vi "Configure Trigger.vi"(0 "VISA resource name":refnum<visa-resource-name>, 5 "Trigger Sequence (1: Output 1)":i32(ring)=1 items=["Output"=1, "Synchronous Source"=2, "Measurement"=3], 7 "Trigger Source (0: Immediate)":i32(ring) items=["Immediate", "Bus", "External", "Phase", "Trigger Out"], 9 "Enable Continuous Triggering (F: Disable)":bool, 11 "error in (no error)":errorcluster, 12 "Trigger Delay (0 s)":dbl format="%#.5g", 13 "Phase Reference (0)":dbl format="%#.4g") -> (4 "VISA resource name out":refnum<visa-resource-name>, 15 "error out":errorcluster)   [LabVIEW 2019, in "Agilent 681x Series.lvlib"]
doc: "Configures the trigger sequences and settings of the instrument."
uses:
  <instrlib>/Agilent 681x Series/Agilent 681x Series.lvlib
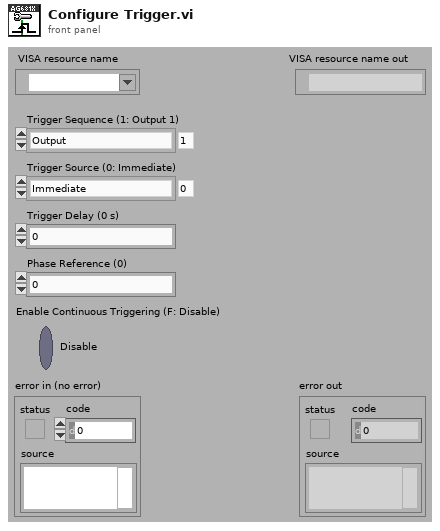
[diagram p1: front panel]
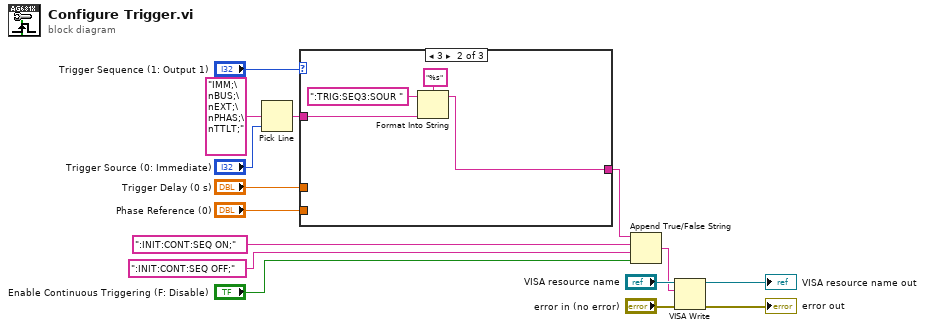
[diagram p0: block diagram]
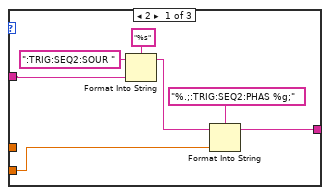
[diagram p2: hidden frame]
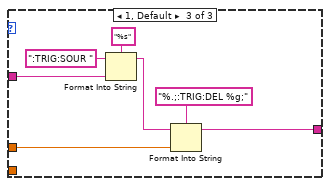
[diagram p3: hidden frame]
diagram:
  n1 = Pick Line(multi-line string="IMM;\nBUS;\nEXT;\nPHAS;\nTTLT;", line index="Trigger Source (0: Immediate)") -> (output string=w10:string)  [unwired: 1 in]
  n2 = case shown="3" "Trigger Sequence (1: Output 1)" {
    tunnel: w10 -> [w18 w24 w32]
    tunnel: "Trigger Delay (0 s)" -> [_ _ w29]
    tunnel: [w16 w23 w27] -> w7
    tunnel: "Phase Reference (0)" -> [w17 _ _]
    frame 2 {
      n3 = Format Into String(format string="%s", initial string=":TRIG:SEQ2:SOUR ", w18) -> (resulting string=w21:string)  [unwired: 1 in, 1 out]
      n4 = Format Into String(format string="%.;:TRIG:SEQ2:PHAS %g;", initial string=w21, w17) -> (resulting string=w16:string)  [unwired: 1 in, 1 out]
    }
    frame 3 {
      n5 = Format Into String(format string="%s", initial string=":TRIG:SEQ3:SOUR ", w24) -> (resulting string=w23:string)  [unwired: 1 in, 1 out]
    }
    frame 1, Default {
      n6 = Format Into String(format string="%s", initial string=":TRIG:SOUR ", w32) -> (resulting string=w30:string)  [unwired: 1 in, 1 out]
      n7 = Format Into String(format string="%.;:TRIG:DEL %g;", initial string=w30, w29) -> (resulting string=w27:string)  [unwired: 1 in, 1 out]
    }
  }
  n8 = Append True/False String(1:"Enable Continuous Triggering (F: Disable)", 2:":INIT:CONT:SEQ OFF;" ("true string"), 3:":INIT:CONT:SEQ ON;" ("true string"), 4:w7) -> (0:w3:string)
  n9 = VISA Write(VISA resource name="VISA resource name", write buffer=w3, error in (no error)="error in (no error)") -> (VISA resource name out=→"VISA resource name out":refnum<visa-resource-name>, error out=→"error out":errorcluster)  [unwired: 1 out]
